vi "currently listening.vi"(11 "connection server in":refnum<class "connection server.lvclass">) -> (3 "listening?":bool)   [LabVIEW 2015, in "connection server.lvclass"]
uses:
  connection server.lvclass
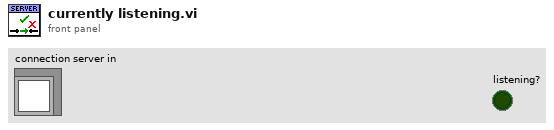
[diagram p1: front panel]
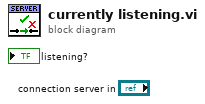
[diagram p0: block diagram]
diagram:
